vi "^AControl.vi"   [LabVIEW 2020]
doc: "Anti-Control Node\n\nCondition for a Controlled Operation. \nThe target gate is applied ONLY if this control qubit is in the |0> state.\n\nBlock Matrix Structure: [[ U, 0], [ 0, 1]] Where U is the target operation."
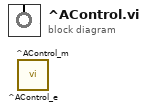
[diagram p0: block diagram]
diagram:
  n1 = call "^AControl_e.vi"() -> ()  [unwired: 14 in, 2 out]
  n2 = call "^AControl_m.vi"() -> ()  [unwired: 14 in, 2 out]
